vi "Add Descendents to Items Map.vi"(8 "error in (no error)":errorcluster, 9 "Order":i32, 11 "Descendents Refs":refnum<vi>[](array[refnum])) -> (0 "error out":errorcluster, 3 "Items":refnum<class "Item.lvclass">[](array[class]))   [LabVIEW 2020, in "VI Properties Editor.lvlib"]
uses:
  VI Properties Editor.lvlib
  Classes/Item/Item.lvclass
  Classes/Support/Item Type.ctl
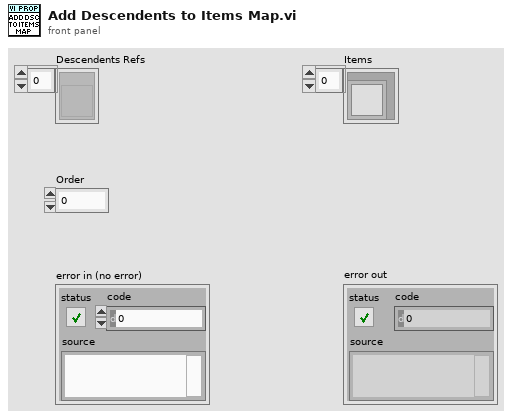
[diagram p1: front panel]
types:
  T1 = typedef "imagedata.ctl" = cluster{"image type":i32, "image depth":i32, "image":u8[], "mask":u8[], "colors":u32[], "Rectangle":cluster{"left":i16, "top":i16, "right":i16, "bottom":i16}}
  T2 = cluster{"Private":T1, "Protected":T1, "Community":T1}
  T3 = typedef "VI Properties Editor.lvlib/Item Type.ctl" = enum16{"Generic", "VI"}
  T4 = enum32{"invalid scope", "public", "private", "protected", "community"}
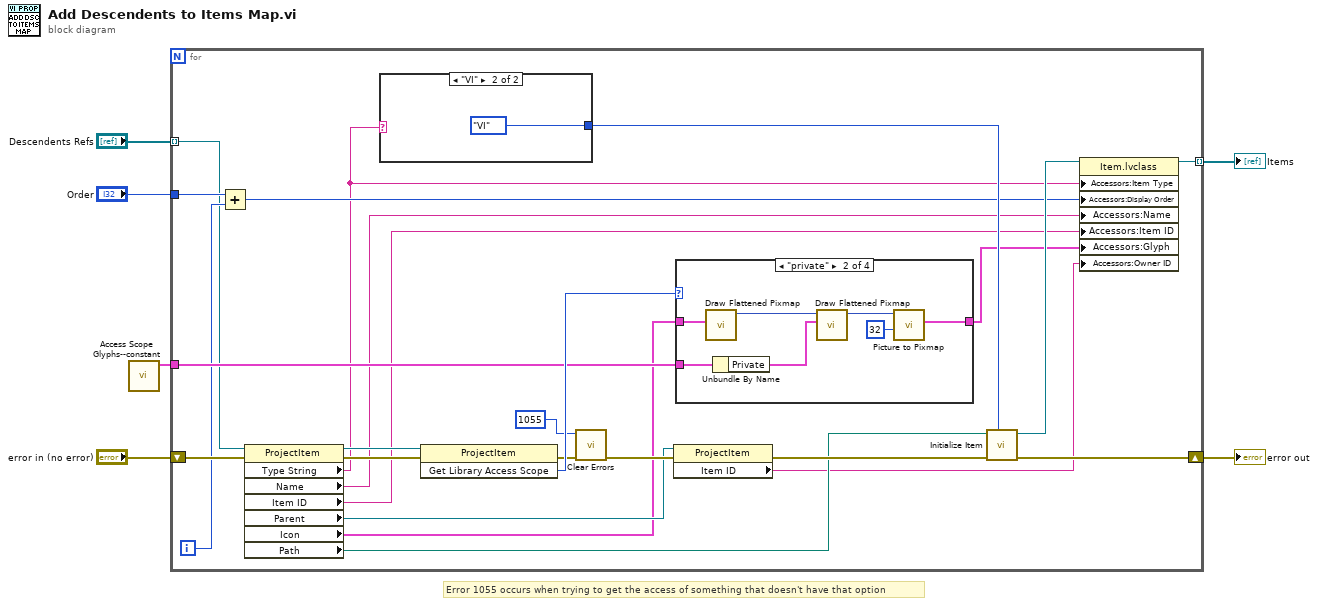
[diagram p0: block diagram]
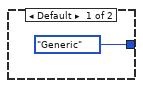
[diagram p2: hidden frame]
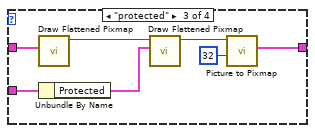
[diagram p4: hidden frame]
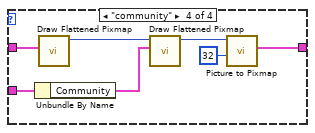
[diagram p5: hidden frame]
diagram:
  # "Error 1055 occurs when trying to get the access of something that doesn't have that option"
  n1 = call "Access Scope Glyphs--constant.vi"() -> ("Access Scope Glyphs"=w2:T2)  [unwired: 11 in]
  n2 = for {
    shift-right: [w13] -> w4
    shift-left: "error in (no error)" -> [w30]
    tunnel: "Descendents Refs" -> [w23] mode=indexing
    tunnel: w2 -> [w26]
    tunnel: "Order" -> [w25]
    tunnel: [w14] -> w1 mode=indexing
    i -> [w24]
    n3 = Add(x=w25, y=w24) -> (x+y=w12:i32)
    n4 = property class="ProjectItem"(reference=w23, error in=w30) -> (reference out=w28:refnum<vi>, error out=w29:errorcluster, "Type String"=w11:string, "Name"=w10:string, "Item ID"=w8:string, "Parent"=w21:refnum<vi>, "Icon"=w20:T1, "Path"=w16:path)
    n5 = case shown="\"VI\"" w11 {
      tunnel: [Item_Type."Generic" ("Item Type") Item_Type."VI" ("Item Type")] -> w17
      frame Default {
      }
      frame "VI" {
      }
    }
    n6 = invoke class="ProjectItem" method="Get Library Access Scope"(reference=w28, error in=w29) -> (error out=w19:errorcluster, "Get Library Access Scope"=w27:T4)  [unwired: 1 in, 1 out]
    n7 = call <vilib>:"Clear Errors.vi"("error in (no error)"=w19, "specific error code to clear (0: all)"=1055) -> ("error out"=w31:errorcluster)  [unwired: 4 in, 1 out]
    n8 = property class="ProjectItem"(reference=w21, error in=w31) -> (error out=w18:errorcluster, "Item ID"=w9:string)  [unwired: 1 out]
    n9 = case shown="\"private\"" w27 {
      tunnel: w26 -> [_ w36 w43 w50]
      tunnel: w20 -> [w34 w41 w48 w55]
      tunnel: [w34 w38 w45 w52] -> w7
      frame "invalid scope", "public" {
      }
      frame "private" {
        n10 = call <vilib>:"Draw Flattened Pixmap.vi"("image data"=w41) -> ("new picture"=w40:picture)  [unwired: 8 in]
        n11 = Unbundle By Name(w36) -> ("Private"=w35:T1)
        n12 = call <vilib>:"Draw Flattened Pixmap.vi"("image data"=w35, "picture"=w40) -> ("new picture"=w39:picture)  [unwired: 7 in]
        n13 = call <vilib>:"Picture to Pixmap.vi"("depth"=32, "picture"=w39) -> ("image data"=w38:T1)  [unwired: 8 in, 1 out]
      }
      frame "protected" {
        n14 = call <vilib>:"Draw Flattened Pixmap.vi"("image data"=w48) -> ("new picture"=w47:picture)  [unwired: 8 in]
        n15 = Unbundle By Name(w43) -> ("Protected"=w42:T1)
        n16 = call <vilib>:"Draw Flattened Pixmap.vi"("image data"=w42, "picture"=w47) -> ("new picture"=w46:picture)  [unwired: 7 in]
        n17 = call <vilib>:"Picture to Pixmap.vi"("depth"=32, "picture"=w46) -> ("image data"=w45:T1)  [unwired: 8 in, 1 out]
      }
      frame "community" {
        n18 = Unbundle By Name(w50) -> ("Community"=w49:T1)
        n19 = call <vilib>:"Draw Flattened Pixmap.vi"("image data"=w55) -> ("new picture"=w54:picture)  [unwired: 8 in]
        n20 = call <vilib>:"Draw Flattened Pixmap.vi"("image data"=w49, "picture"=w54) -> ("new picture"=w53:picture)  [unwired: 7 in]
        n21 = call <vilib>:"Picture to Pixmap.vi"("depth"=32, "picture"=w53) -> ("image data"=w52:T1)  [unwired: 8 in, 1 out]
      }
    }
    n22 = call "Initialize Item.vi"("Item Type"=w17, "error in (no error)"=w18, "Path"=w16) -> ("error out"=w13:errorcluster, "Item"=w15:refnum<class "Item.lvclass">)  [unwired: 7 in]
    n23 = property class="Item.lvclass"(reference=w15, "Accessors:Item Type"=w11, "Accessors:Display Order"=w12, "Accessors:Name"=w10, "Accessors:Item ID"=w8, "Accessors:Glyph"=w7, "Accessors:Owner ID"=w9) -> (reference out=w14:refnum<class "Item.lvclass">)  [unwired: 1 in, 1 out]
  }
  "error out" <- w4
  "Items" <- w1
